vi "PA Get Power Data.vi"(7 "BufferSize":i32, 9 "pPower":dbl[](array[numeric])=array[4097 elements], 10 "Channel":i32, 11 "DevHandle":i32) -> (1 "pPower out":dbl[](array[numeric]), 3 "function return":i32)   [LabVIEW 2010, in "power_analyzer.lvlib"]
doc: "int WINAPI PA_GetPowerData(int DevHandle,int Channel,double *pPower,int BufferSize);"
uses:
  power_analyzer.lvlib
  USB2XXX/trunk/USB2XXX/USB2XXX/vs2010/Release/USB2XXX.dll
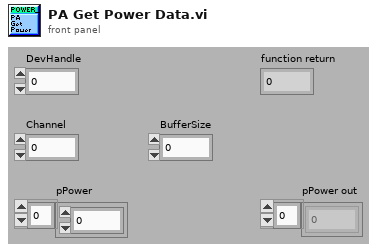
[diagram p1: front panel]
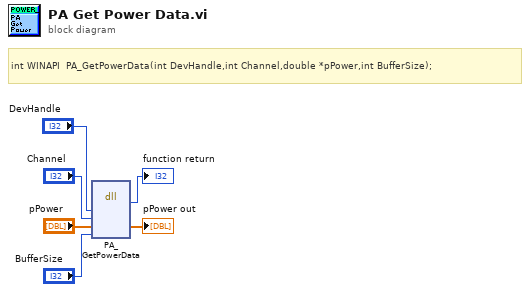
[diagram p0: block diagram]
diagram:
  # "int WINAPI  PA_GetPowerData(int DevHandle,int Channel,double *pPower,int BufferSize);"
  n1 = dll-call lib="E:/Projects/USB2XXX/trunk/USB2XXX/USB2XXX/vs2010/Release/USB2XXX.*" fn="PA_GetPowerData"("DevHandle"="DevHandle", "Channel"="Channel", "pPower"="pPower", "BufferSize"="BufferSize") -> (→"function return":i32, "pPower"=→"pPower out":dbl[])  [unwired: 6 in, 2 out]
